vi "Preallocated A x B  (DBL).vi"(9 "Preallocated A x B":T1, 10 "B":T1, 11 "A":T1) -> (0 "error":i32, 3 "A x B":T1)   [LabVIEW 2018, in "NI_AALPro.lvlib"]
doc: "Performs the multiplication of two input matrices or an input matrix and an input vector. The data types you wire to the <B>A</B> and <B>B</B> inputs determine the polymorphic instance to use."
uses:
  NI_AALPro.lvlib
  RealMatrix.ctl
  <resource>/lvanlys.dll
  NI_Matrix.lvlib
panel:
  # "Preallocated A x B"
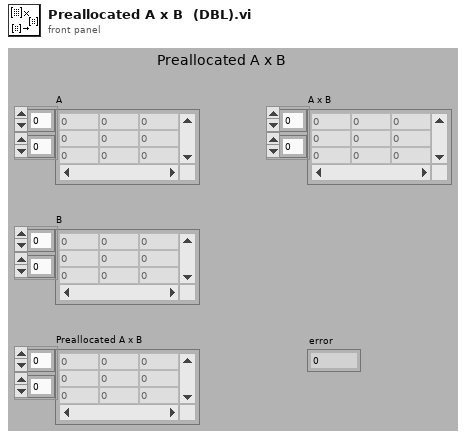
[diagram p1: front panel]
types:
  T1 = typedef "NI_Matrix.lvlib/RealMatrix.ctl" = dbl[][]
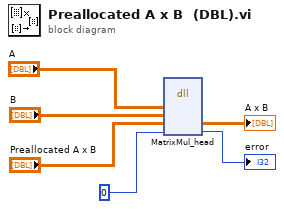
[diagram p0: block diagram]
diagram:
  n1 = dll-call lib="C:/Program Files (x86)/National Instruments/LabVIEW 2018/resource/lvanlys.*" fn="MatrixMul_head"("aHandle"="A", "bHandle"="B", "A x B"="Preallocated A x B", "dsperr"=0) -> ("A x B"=→"A x B":T1, "dsperr"=→"error":i32)  [unwired: 6 in, 2 out]
